vi "Delete Batch .vi"(7 "Batch Data 3":T1, 8 "error in (no error) 5":errorcluster, 9 "Module Number":dbl, 10 "Primery key names":string[](array[string]), 11 "Primery key last values":string[](array[string])) -> (3 "Sucess ?":bool)   [LabVIEW 2015, in "Copy of Untitled Library 1.lvlib"]
uses:
  Copy of Untitled Library 1.lvlib
  Controls/Caller Queue Control .ctl
  Controls/Control 1.ctl
  <userlib>/origin_lib_main/db_interface/DB Operations Enum.ctl
  Controls/Enum Constant.ctl
  <userlib>/origin_lib_main/db_interface/DB Interface.lvlib
panel:
  in  "Cluster":T2
  out "format string 2":string
  out "error out":errorcluster
  out "concatenated string":string
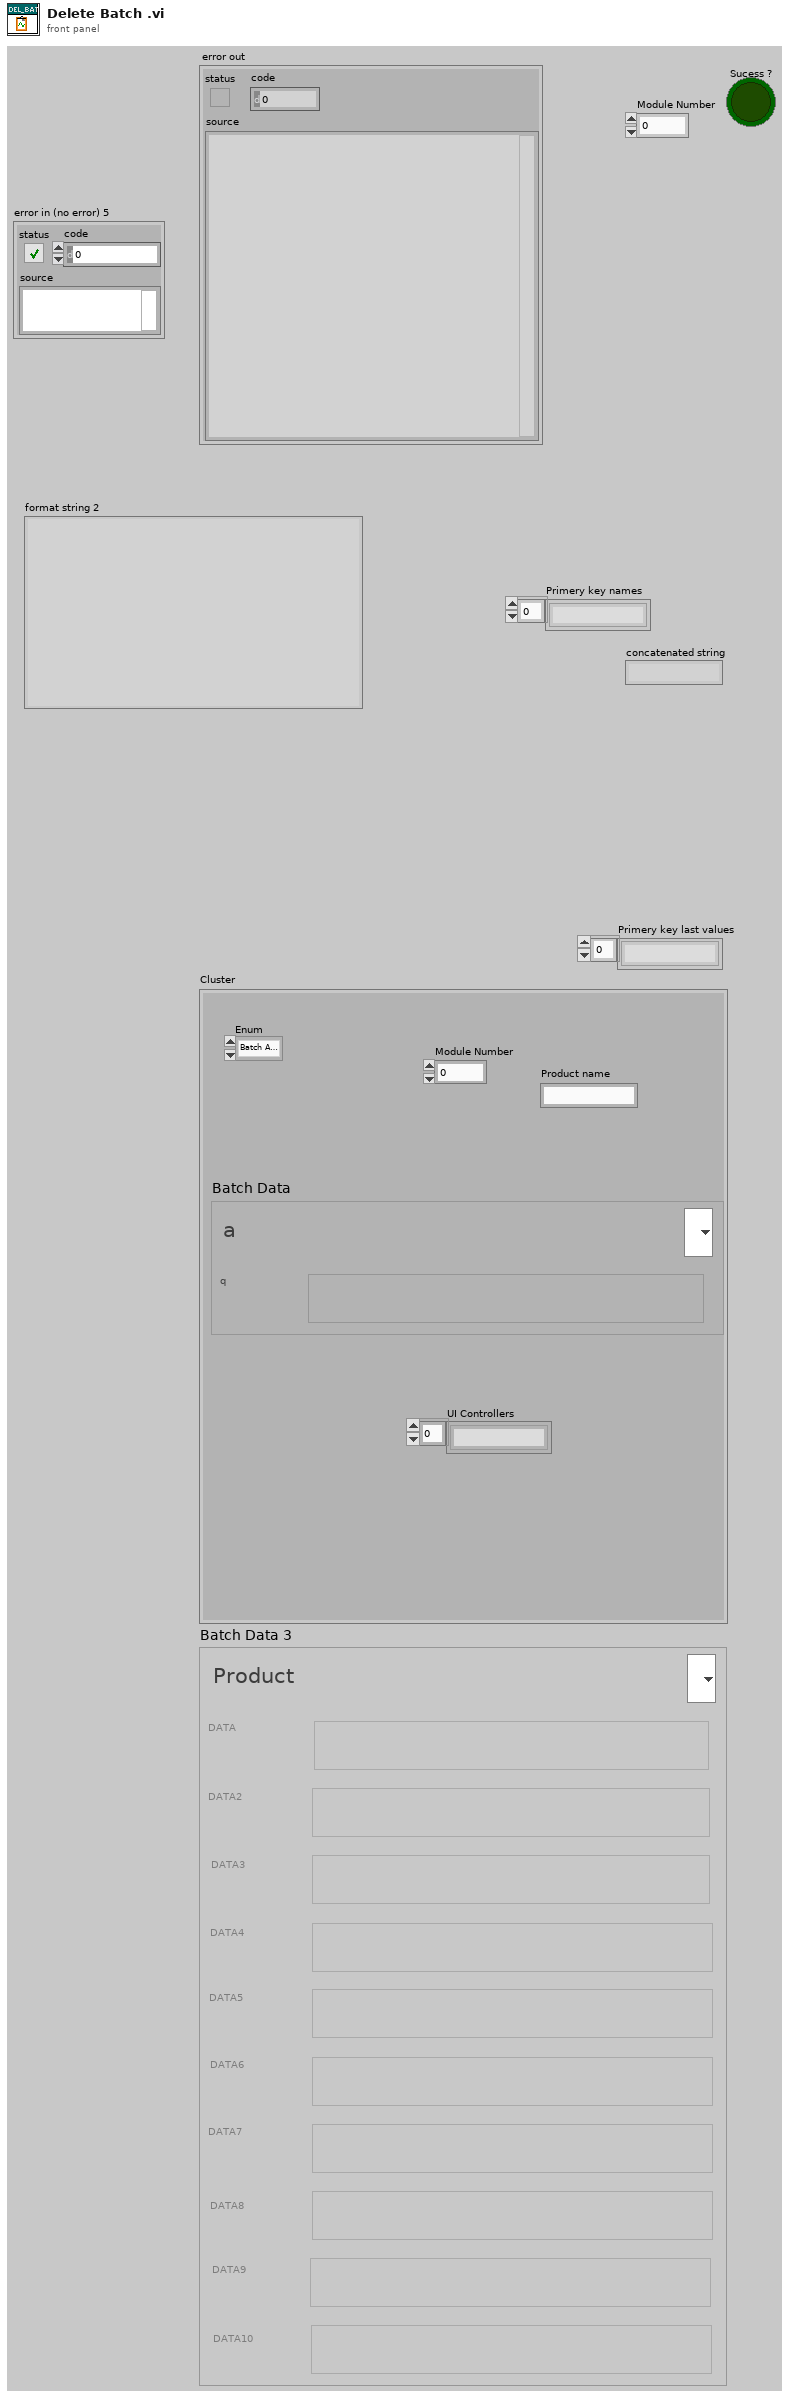
[diagram p1: front panel]
types:
  T1 = typedef "Copy of Untitled Library 1.lvlib/Control 1.ctl" = cluster{"DATA":string, "DATA 2":string, "DATA 3":string, "DATA 4":string, "DATA 5":string, "DATA 6":string, "DATA 7":string, "DATA 8":string, "DATA 9":string, "DATA 10":string, "Product":string}
  T2 = typedef "Caller Queue Control .ctl" = cluster{"Enum":enum16{"Batch Added", "Batch Deleted", "Batch Opened", "Batch Closed", "Batch Edited", "new Product Added", "Product deleted "}, "Batch Data 3":T1, "UI Controllers":string[], "Product name":string, "Module Number":dbl}
  T3 = typedef "Enum Constant.ctl" = enum16{"Init", "Read", "Write"}
  T4 = typedef "DB Interface.lvlib/DB Operations Enum.ctl" = enum16{"Select", "Update", "Insert", "Delete", "Fetch SQL Query", "Execute SQL Query", "Drop Table", "List Tables"}
  T5 = typedef "FGV Data.ctl" = T6[]
  T6 = typedef "FGV Cluster Data.ctl" = cluster{"Manual/Automatic":bool, "UI Controllers ":string[], "UI Primery Key ":dbl[], "Caller Queue & MSG":T7, "Module ID":dbl, "DB Reference In":T8, "Products Columns":string[], "Cluster":cluster{"Delete Product":enum8{"Enabled", "Disabled", "Disabled and Grayed Out"}, "Add Product ":enum8{"Enabled", "Disabled", "Disabled and Grayed Out"}, "EDIT BATCH":enum8{"Enabled", "Disabled", "Disabled and Grayed Out"}, "Open Batch ":enum8{"Enabled", "Disabled", "Disabled and Grayed Out"}, "Close Batch":enum8{"Enabled", "Disabled", "Disabled and Grayed Out"}, "Delete Batch":enum8{"Enabled", "Disabled", "Disabled and Grayed Out"}, "Add Batch ":enum8{"Enabled", "Disabled", "Disabled and Grayed Out"}}}
  T7 = typedef "Queue and Caller MSG.ctl" = cluster{"Caller Queue":refnum<queue>, "Caller MSG":string}
  T8 = typedef "NI_Database_API.lvlib/Conn ObjectReference.ctl" = refnum<k1>
  T9 = enum16{"Batch Added", "Batch Deleted", "Batch Opened", "Batch Closed", "Batch Edited", "new Product Added", "Product deleted "}
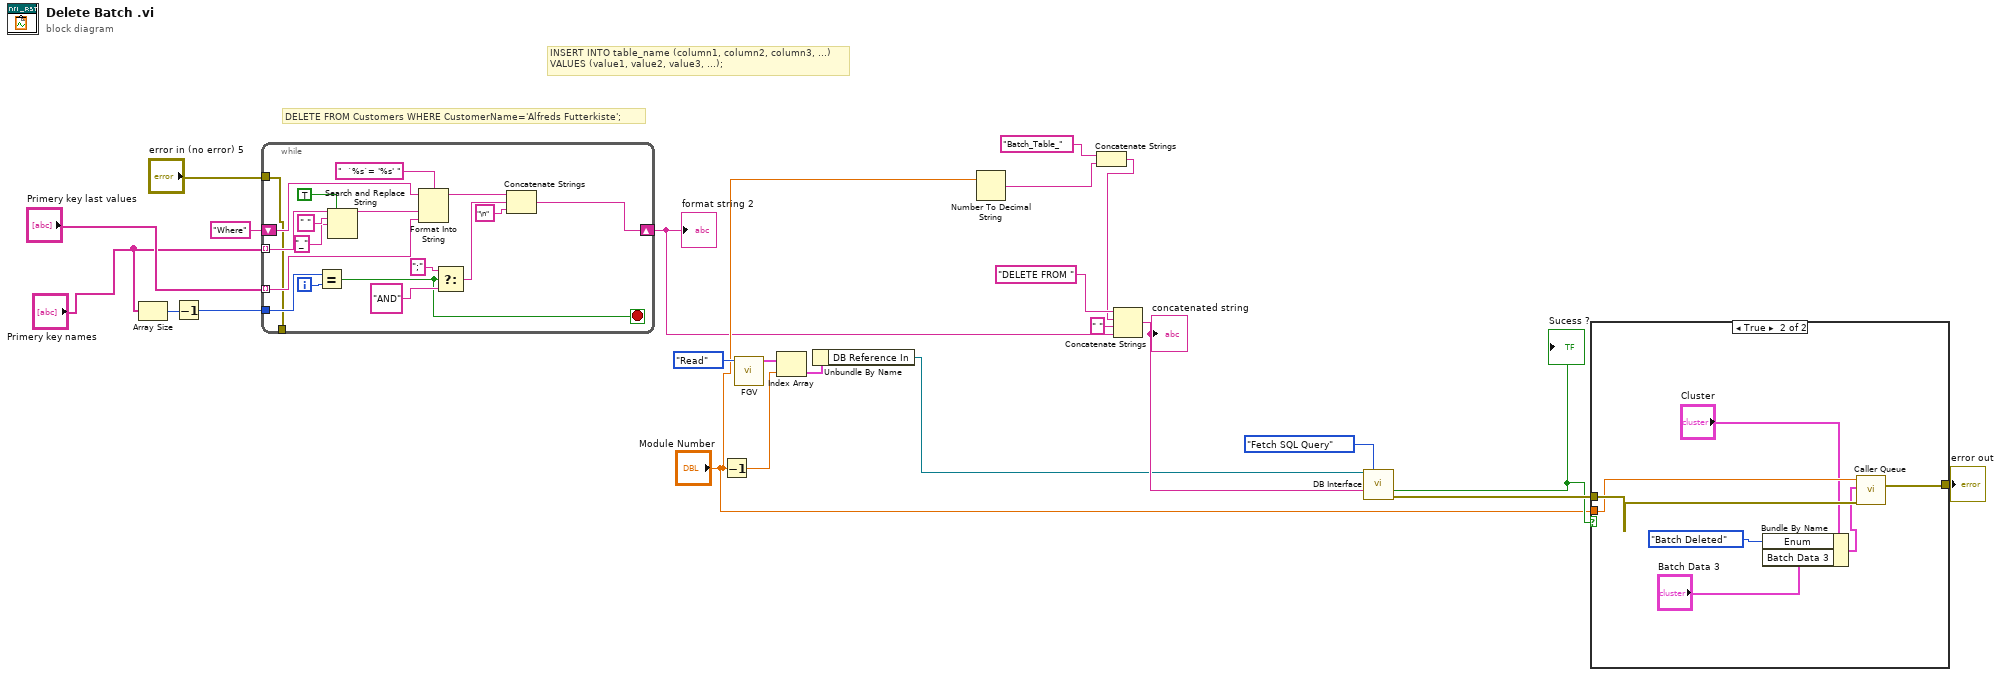
[diagram p0: block diagram]
diagram:
  # "DELETE FROM Customers WHERE CustomerName='Alfreds Futterkiste';"
  # "INSERT INTO table_name (column1, column2, column3, ...)\nVALUES (value1, value2, value3, ...);"
  n1 = Array Size(array="Primery key names") -> (size(s)=w16:i32)
  n2 = Decrement(x=w16) -> (x-1=w15:i32)
  n3 = while {
    shift-right: [w28] -> w1
    shift-left: "Where" ("format string") -> [w40]
    tunnel: w15 -> [w34]
    tunnel: "Primery key names" -> [w29] mode=indexing
    tunnel: "Primery key last values" -> [w26] mode=indexing
    tunnel: [w24] -> _
    tunnel: "error in (no error) 5" -> [w24]
    i -> [w35]
    stop <- w25 stop-if-true
    n4 = Equal?(x=w34, y=w35) -> (x = y?=w25:bool)
    n5 = Search and Replace String(replace all?=TRUE ("replace all? (F)"), input string=w29, search string=" ", replace string="_" ("replace string (\"\")")) -> (result string=w30:string)  [unwired: 4 in, 3 out]
    n6 = Format Into String(format string="  `%s`= '%s' ", initial string=w40, w30, w26) -> (resulting string=w39:string)  [unwired: 1 in, 1 out]
    n7 = Select(t=";", s=w25, f="AND") -> (s? t:f=w36:string)
    n8 = Concatenate Strings(w39, w36, "\n" ("string")) -> (w28:string)
  }
  "format string 2" <- w1
  n9 = Decrement(x="Module Number") -> (x-1=w8:dbl)
  n10 = call "FGV.vi"("Enum"=Enum_Constant."Read") -> ("Read Data"=w10:T5)  [unwired: 9 in, 1 out]
  n11 = Index Array(array=w10, index=w8) -> (element=w9:T6)
  n12 = Unbundle By Name(w9) -> ("DB Reference In"=w7:T8)
  n13 = Number To Decimal String(number="Module Number") -> (decimal integer string=w21:string)  [unwired: 1 in]
  n14 = Concatenate Strings("Batch_Table_" ("string"), w21) -> (w20:string)
  n15 = Concatenate Strings("DELETE FROM " ("string"), w20, " " ("string"), w1) -> (w18:string)
  "concatenated string" <- w18
  n16 = call <userlib>:"DB Interface.vi"("DB Ref In"=w7, "Operation"=DB_Operations_Enum."Fetch SQL Query", "SQL Query"=w18) -> ("Sucess ?"=w3:bool, "error out"=w5:errorcluster)  [unwired: 9 in, 2 out]
  "Sucess ?" <- w3
  n17 = case shown="True" w3 {
    tunnel: w5 -> [w42 w49]
    tunnel: [w42 w48] -> w4
    tunnel: "Module Number" -> [_ w47]
    frame False {
    }
    frame True {
      n18 = Bundle By Name(cluster="Cluster", "Enum"=T9."Batch Deleted", "Batch Data 3"="Batch Data 3") -> (w43:T2)
      n19 = call "Caller Queue .vi"("error in (no error)"=w49, "Cluster"=w43, "Module Number  3"=w47) -> ("error out"=w48:errorcluster)  [unwired: 8 in]
    }
  }
  "error out" <- w4
